vi "мажоритарный 5.vi"() -> ()   [LabVIEW 2013]
panel:
  out "result":u32
  in  "5":dbl
  in  "4":dbl
  in  "3":dbl
  in  "2":dbl
  in  "1":dbl
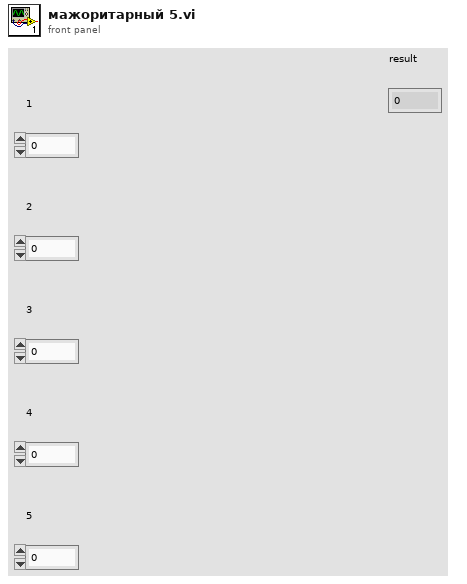
[diagram p1: front panel]
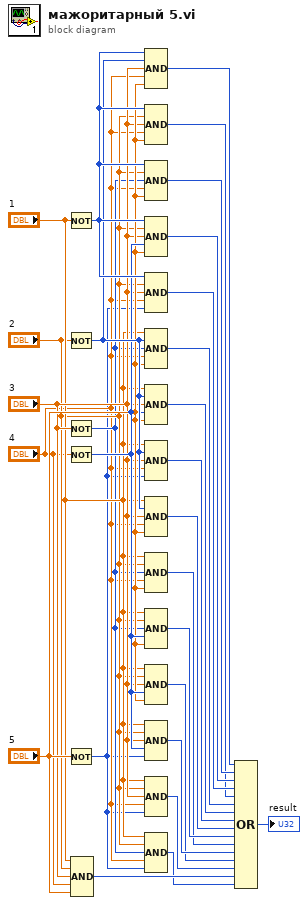
[diagram p0: block diagram]
diagram:
  n1 = Not(x="1") -> (.not. x?=w27:u32)
  n2 = Not(x="2") -> (.not. x?=w26:u32)
  n3 = Not(x="3") -> (.not. x?=w4:u32)
  n4 = Not(x="4") -> (.not. x?=w25:u32)
  n5 = Not(x="5") -> (.not. x?=w2:u32)
  n6 = Compound Arithmetic op=AND("1", "2", "3", "4", "5") -> (w8:i32)
  n7 = Compound Arithmetic op=AND(w27, w26, "3", "4", "5") -> (w22:i32)
  n8 = Compound Arithmetic op=AND(w27, "2", "3", "4", "5") -> (w18:i32)
  n9 = Compound Arithmetic op=AND(w27, "2", w4, "4", "5") -> (w21:i32)
  n10 = Compound Arithmetic op=AND(w27, "2", "3", w25, "5") -> (w20:i32)
  n11 = Compound Arithmetic op=AND(w27, "2", "3", "4", w2) -> (w19:u32)
  n12 = Compound Arithmetic op=AND("1", w26, w4, "4", "5") -> (w17:i32)
  n13 = Compound Arithmetic op=AND("1", w26, "3", w25, "5") -> (w16:i32)
  n14 = Compound Arithmetic op=AND("1", w26, "3", "4", w2) -> (w15:u32)
  n15 = Compound Arithmetic op=AND("1", w26, "3", "4", "5") -> (w14:i32)
  n16 = Compound Arithmetic op=AND("1", "2", w4, "4", "5") -> (w12:i32)
  n17 = Compound Arithmetic op=AND("1", "2", w4, w25, "5") -> (w13:i32)
  n18 = Compound Arithmetic op=AND("1", "2", "3", w25, "5") -> (w10:i32)
  n19 = Compound Arithmetic op=AND("1", "2", "3", w25, w2) -> (w11:u32)
  n20 = Compound Arithmetic op=AND("1", "2", "3", "4", w2) -> (w9:u32)
  n21 = Compound Arithmetic op=AND("1", "2", w4, "4", w2) -> (w1:u32)
  n22 = Compound Arithmetic op=OR(w22, w21, w20, w19, w18, w17, w16, w15, w14, w13, w12, w11, w10, w9, w8, w1) -> (→"result":u32)
